vi "Write Offset.vi"(8 "error in (no error)":errorcluster, 10 "Offset":dbl, 11 "Composite Waveform in":refnum<class "Composite Waveform.lvclass">) -> (0 "error out":errorcluster, 3 "Composite Waveform out":refnum<class "Composite Waveform.lvclass">)   [LabVIEW 2020, in "Composite Waveform.lvclass"]
uses:
  Composite Waveform.lvclass
  Composite Waveform.lvclass/Composite Waveform.ctl
  Analog Waveform/Analog Waveform.lvclass
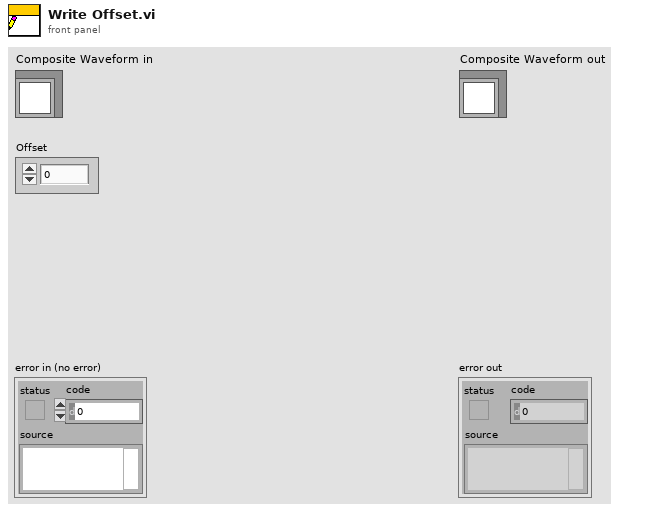
[diagram p1: front panel]
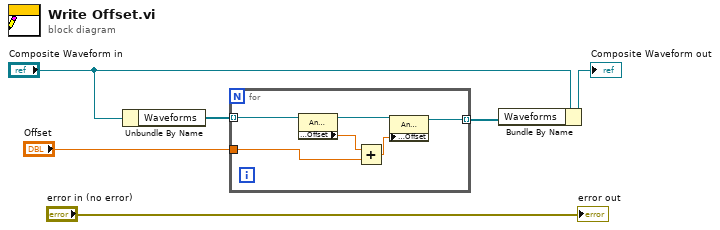
[diagram p0: block diagram]
diagram:
  n1 = Unbundle By Name("Composite Waveform in") -> ("Waveforms"=w3:refnum<class "Analog Waveform.lvclass">[])
  n2 = for {
    tunnel: w3 -> [w12] mode=indexing
    tunnel: [w11] -> w2 mode=indexing
    tunnel: "Offset" -> [w10]
    n3 = property class="Analog Waveform.lvclass"(reference=w12) -> (reference out=w9:refnum<class "Analog Waveform.lvclass">, "Member Accessors:Offset"=w7:dbl)  [unwired: 1 in, 1 out]
    n4 = Add(x=w7, y=w10) -> (x+y=w8:dbl)
    n5 = property class="Analog Waveform.lvclass"(reference=w9, "Member Accessors:Offset"=w8) -> (reference out=w11:refnum<class "Analog Waveform.lvclass">)  [unwired: 1 in, 1 out]
  }
  n6 = Bundle By Name(cluster="Composite Waveform in", "Waveforms"=w2) -> (→"Composite Waveform out":refnum<class "Composite Waveform.lvclass">)
  "error out" <- "error in (no error)"
